vi "SetMenuItemsPositionAndBounds.vi"(8 "error in (no error)":errorcluster, 11 "menu in":refnum<class "menu.lvclass">) -> (0 "error out":errorcluster, 3 "menu out":refnum<class "menu.lvclass">)   [LabVIEW 2009, in "menu.lvclass"]
uses:
  menu.lvclass
  menu.lvclass/menu.ctl
  Menu Item/menu item.lvclass
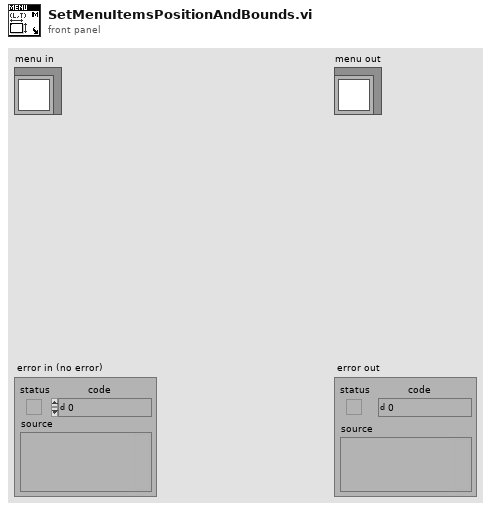
[diagram p1: front panel]
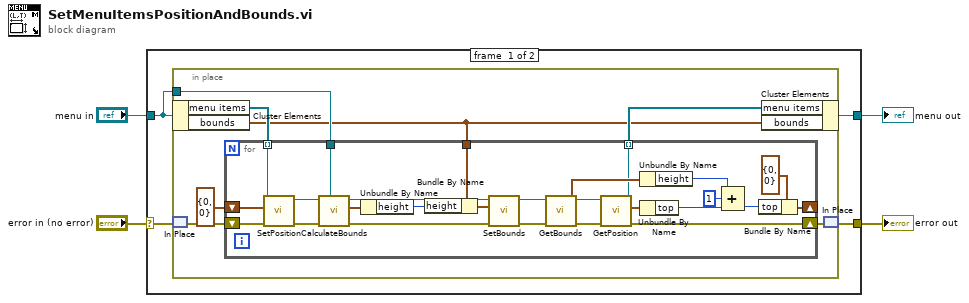
[diagram p0: block diagram]
diagram:
  n1 = case shown="No Error" "error in (no error)" {
    selector: "error in (no error)" -> [w8 w43]
    tunnel: [w7 w43] -> w1
    tunnel: [w5 w42] -> w3
    tunnel: "menu in" -> [w6 w42]
    frame #0 {
      n2 = in-place {
        in-place-border: w6 -> [w12]
        n3 = in-place-cluster #1(w6) -> ("menu items"=w15:refnum<class "menu item.lvclass">[], "bounds"=w9:cluster{"width":u32, "height":u32})
        n4 = in-place-match #2(w8) -> (w11:errorcluster)
        n5 = for {
          shift-right: [w34] -> w13
          shift-left: w11 -> [w35]
          tunnel: w12 -> [w33]
          shift-right: [w29] -> _
          shift-left: cluster{"left":u32, "top":u32} {"left"=0, "top"=0} ("position") -> [w32]
          tunnel: w15 -> [w24] mode=indexing
          tunnel: [w23] -> w14 mode=indexing
          tunnel: w9 -> [w19]
          n6 = call-dynamic "SetPosition.vi"("error in (no error)"=w35, "position"=w32, "menu item in"=w24) -> ("error out"=w37:errorcluster, "menu item out"=w36:refnum<class "menu item.lvclass">)  [unwired: 7 in]
          n7 = call-dynamic "CalculateBounds.vi"("menu in"=w33, "error in (no error)"=w37, "menu item in"=w36) -> ("error out"=w39:errorcluster, "bounds"=w17:cluster{"width":u32, "height":u32}, "menu item out"=w38:refnum<class "menu item.lvclass">)  [unwired: 6 in]
          n8 = Unbundle By Name(w17) -> ("height"=w16:u32)
          n9 = Bundle By Name(cluster=w19, "height"=w16) -> (w18:cluster{"width":u32, "height":u32})
          n10 = call-dynamic "SetBounds.vi"("error in (no error)"=w39, "bounds"=w18, "menu item in"=w38) -> ("error out"=w26:errorcluster, "menu item out"=w25:refnum<class "menu item.lvclass">)  [unwired: 7 in]
          n11 = call-dynamic "GetBounds.vi"("error in (no error)"=w26, "menu item in"=w25) -> ("error out"=w41:errorcluster, "bounds"=w27:cluster{"width":u32, "height":u32}, "menu item out"=w40:refnum<class "menu item.lvclass">)  [unwired: 7 in]
          n12 = call-dynamic "GetPosition.vi"("error in (no error)"=w41, "menu item in"=w40) -> ("error out"=w34:errorcluster, "position"=w28:cluster{"left":u32, "top":u32}, "menu item out"=w23:refnum<class "menu item.lvclass">)  [unwired: 7 in]
          n13 = Unbundle By Name(w27) -> ("height"=w20:u32)
          n14 = Unbundle By Name(w28) -> ("top"=w21:u32)
          n15 = Compound Arithmetic op=ADD(w20, u32 1 ("value"), w21) -> (w30:u32)
          n16 = Bundle By Name(cluster=cluster{"left":u32, "top":u32} {"left"=0, "top"=0} ("position"), "top"=w30) -> (w29:cluster{"left":u32, "top":u32})
        }
        n17 = in-place-cluster #1("menu items"=w14, "bounds"=w9) -> (w5:refnum<class "menu.lvclass">)
        n18 = in-place-match #2(w13) -> (w7:errorcluster)
      }
    }
    frame #1 {
    }
  }
  "menu out" <- w3
  "error out" <- w1
